vi "Test Sessions.vi"() -> ()   [LabVIEW 2020]
uses:
  lv-http-server/HTTP Server/Trace Log.ctl
  lv-http-server/HTTP Server/Trace Item.ctl
  lv-http-server/HTTP Server/Processing Step.ctl
  lv-http-util/HTTP Utils/Method.ctl
  Test Sessions Controller/Test Sessions Controller.lvclass
  C:/dev/lv20CE/relink/lv-http-server/HTTP Server/Handler/Handler.lvclass
  lv-http-server/HTTP Server/Server/Add Connection Handler.vi
  lv-http-server/HTTP Server/Server/Add Request Handler.vi
  lv-http-server/HTTP Server/Server/Add Route Handler.vi
  lv-http-server/HTTP Server/Server/Add Controller Handler.vi
  lv-http-server/HTTP Server/Server/Add Controller.vi
  lv-http-server/HTTP Server/Server/Add Response Handler.vi
  lv-http-server/HTTP Server/Server/Add Complete Handler.vi
  lv-http-server/HTTP Server/Server/Add Exception Handler.vi
  lv-http-server/HTTP Server/Connection Handler/Connection Handler.lvclass
  lv-http-server/HTTP Server/Request Handler/Request Handler.lvclass
  lv-http-server/HTTP Server/Route Handler/Route Handler.lvclass
  lv-http-server/HTTP Server/Controller Handler/Controller Handler.lvclass
  lv-http-server/HTTP Server/Controller/Controller.lvclass
  lv-http-server/HTTP Server/Response Handler/Response Handler.lvclass
  lv-http-server/HTTP Server/Complete Handler/Complete Handler.lvclass
  lv-http-server/HTTP Server/Exception Handler/Exception Handler.lvclass
  lv-http-server/HTTP Server/Server/Server.lvclass
  lv-http-server/HTTP Server/Handler/Handler.lvclass
  lv-http-server/HTTP Server/Session/Session.lvclass
  lv-http-server/HTTP Server/RequestTraceLog/RequestTraceLog.lvclass
  lv-http-server/HTTP Server/HTTP Server.lvlib
  lv-http-util/HTTP Utils/HTTP Utils.lvlib
panel:
  in  "Refresh Traces":bool
  out "Traces":T1[](array[typedef]) {"Sending" format="%_6f"; "Expires" format="%<%X %x>T"; "Created" format="%<%X %x>T"; "Waiting" format="%_6f"; "Parsing" format="%_6f"; "Processing" format="%_6f"; "Items"."Time" format="%.6f"; "Items"."Duration" format="%.6f"}
  # "Request"
  # "Response"
  # "Session"
  # "Auth"
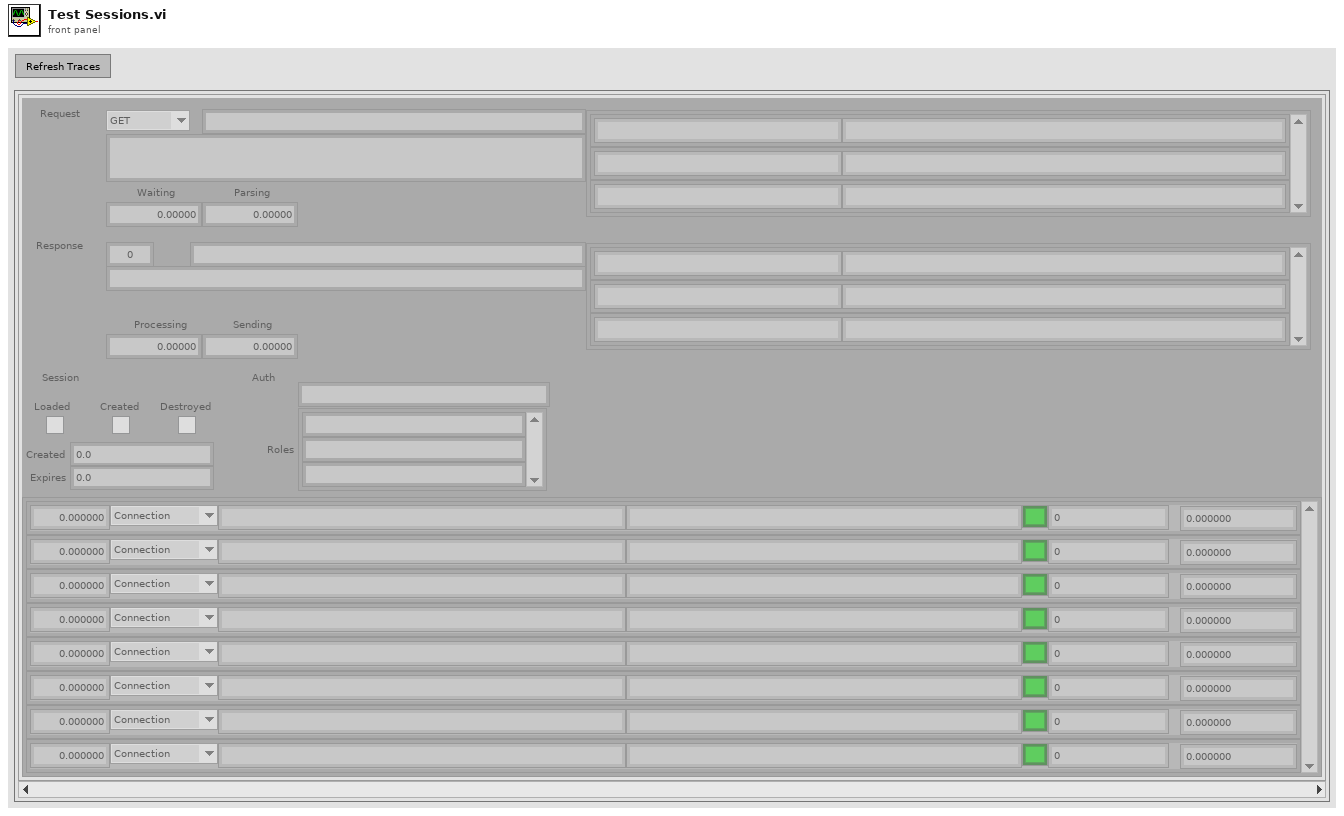
[diagram p1: front panel]
types:
  T1 = typedef "HTTP Server.lvlib/Trace Log.ctl" = cluster{"Items":T2[], "Client":string, "Target":string, "Response Type":string, "Processing":dbl, "Status":u16, "Method":T4, "Content Type":string, "Request Headers":cluster{"Name":string, "Value":string}[], "Parsing":dbl, "Waiting":dbl, "Identity":string, "Loaded":bool, "Created":bool, "Destroyed":bool, "Response Headers":cluster{"Name":string, "Value":string}[], "Created":dbl, "Expires":dbl, "Roles":string[], "Sending":dbl}
  T2 = typedef "HTTP Server.lvlib/Trace Item.ctl" = cluster{"Duration":dbl, "Step":T3, "Class":string, "Info":string, "Status":bool, "Code":i32, "Time":dbl}
  T3 = typedef "HTTP Server.lvlib/Processing Step.ctl" = enum16{"Connection", "Request", "Routing", "Controller Init", "Controller", "Response", "Complete", "Exception"}
  T4 = typedef "HTTP Utils.lvlib/Method.ctl" = enum16{"GET", "HEAD", "POST", "PUT", "DELETE", "CONNECT", "OPTIONS", "TRACE", "PATCH"}
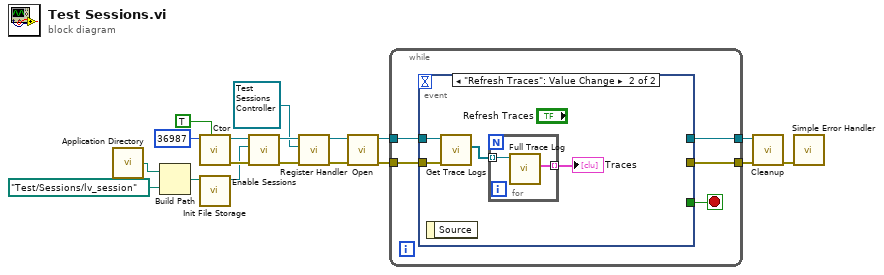
[diagram p0: block diagram]
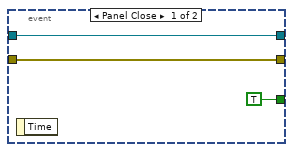
[diagram p2: hidden frame]
diagram:
  n1 = call <vilib>:"Application Directory.vi"() -> ("Application Directory"=w14:path)
  n2 = Build Path(base path=w14, name or relative path=path "Test/Sessions/lv_session") -> (appended path=w12:path)
  n3 = call "Ctor.vi"("Debug (F)"=TRUE, "HTTP Port (80)"=u16 36987 ("Port (8080)")) -> ("error out"=w16:errorcluster, "Server out"=w15:refnum<class "Server.lvclass">)  [unwired: 8 in]
  n4 = call "Init File Storage.vi"("Session Storage Folder"=w12) -> ("Session out"=w11:refnum<class "Session.lvclass">)  [unwired: 9 in, 1 out]
  n5 = call "Enable Sessions.vi"("error in (no error)"=w16, "Session Implementation"=w11, "Server in"=w15) -> ("error out"=w8:errorcluster, "Server out"=w10:refnum<class "Server.lvclass">)  [unwired: 7 in]
  n6 = call "Register Handler.vi"("error in (no error)"=w8, "Handler"=refnum<class "Test Sessions Controller.lvclass"> refnum ("Test Sessions Controller.lvclass"), "Server in"=w10) -> ("error out"=w6:errorcluster, "Server out"=w7:refnum<class "Server.lvclass">)  [unwired: 7 in]
  n7 = call "Open.vi"("error in (no error)"=w6, "Server in"=w7) -> ("error out"=w4:errorcluster, "Server out"=w5:refnum<class "Server.lvclass">)  [unwired: 8 in]
  n8 = while {
    tunnel: w5 -> [w23]
    tunnel: w4 -> [w22]
    tunnel: [w20] -> w3
    tunnel: [w19] -> w2
    stop <- w21 stop-if-true
    n9 = event shown="[1] \"Refresh Traces\": Value Change" {
      selector: _ -> [_ _]
      dyn-events: _ -> [_ _]
      timeout: _ -> [_ _]
      tunnel: w23 -> [w25 w30]
      tunnel: w22 -> [w24 w29]
      tunnel: [TRUE _] -> w21
      tunnel: [w25 _] -> w20
      tunnel: [w24 _] -> w19
      event Panel Close {
        n10 = event-data() -> ()  [unwired: 1 in, 1 out]
      }
      event "Refresh Traces": Value Change {
        n11 = event-data() -> ()  [unwired: 1 in, 1 out]
        n12 = call "Get Trace Logs.vi"("error in (no error)"=w29, "Server in"=w30) -> ("Trace Logs"=w28:refnum<class "RequestTraceLog.lvclass">[])  [unwired: 7 in, 2 out]
        n13 = for {
          tunnel: w28 -> [w32] mode=indexing
          tunnel: [w31] -> w27 mode=indexing
          n14 = call "Full Trace Log.vi"("RequestTraceLog in"=w32) -> ("Trace Log"=w31:T1)  [unwired: 8 in, 2 out]
        }
        "Traces" <- w27
      }
    }
  }
  n15 = call "Cleanup.vi"("error in (no error)"=w2, "Server in"=w3) -> ("error out"=w1:errorcluster)  [unwired: 9 in]
  n16 = call <vilib>:"Simple Error Handler.vi"("error in (no error)"=w1) -> ()  [unwired: 4 in, 5 out]
